vi "Run.vi"(8 "error in (no error)":errorcluster, 11 "Opctics in":refnum<class "Opt_Continuous.lvclass">) -> (0 "error out":errorcluster, 3 "Opt_Continuous out":refnum<class "Opt_Continuous.lvclass">)   [LabVIEW 2018, in "Opt_Continuous.lvclass"]
uses:
  Opt_Continuous.lvclass
  C:/Users/observer/Desktop/Sparc4GUI/SPARC4_GUI/Device/Optics/Optics.lvclass
  Optics.lvclass/Optics.ctl
  Optics.lvclass
  StateMachine/State Machine.lvclass
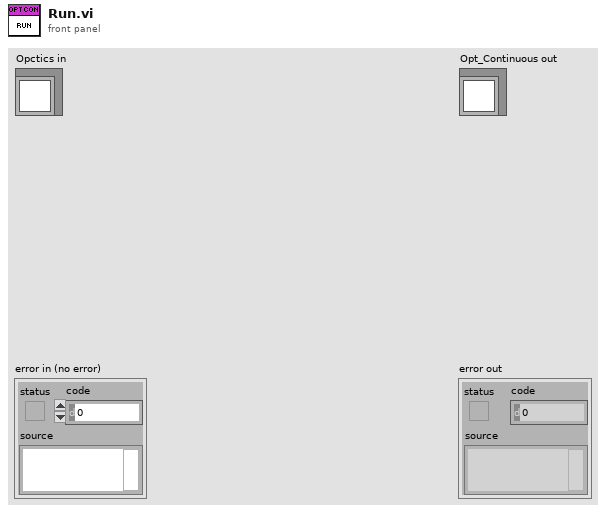
[diagram p1: front panel]
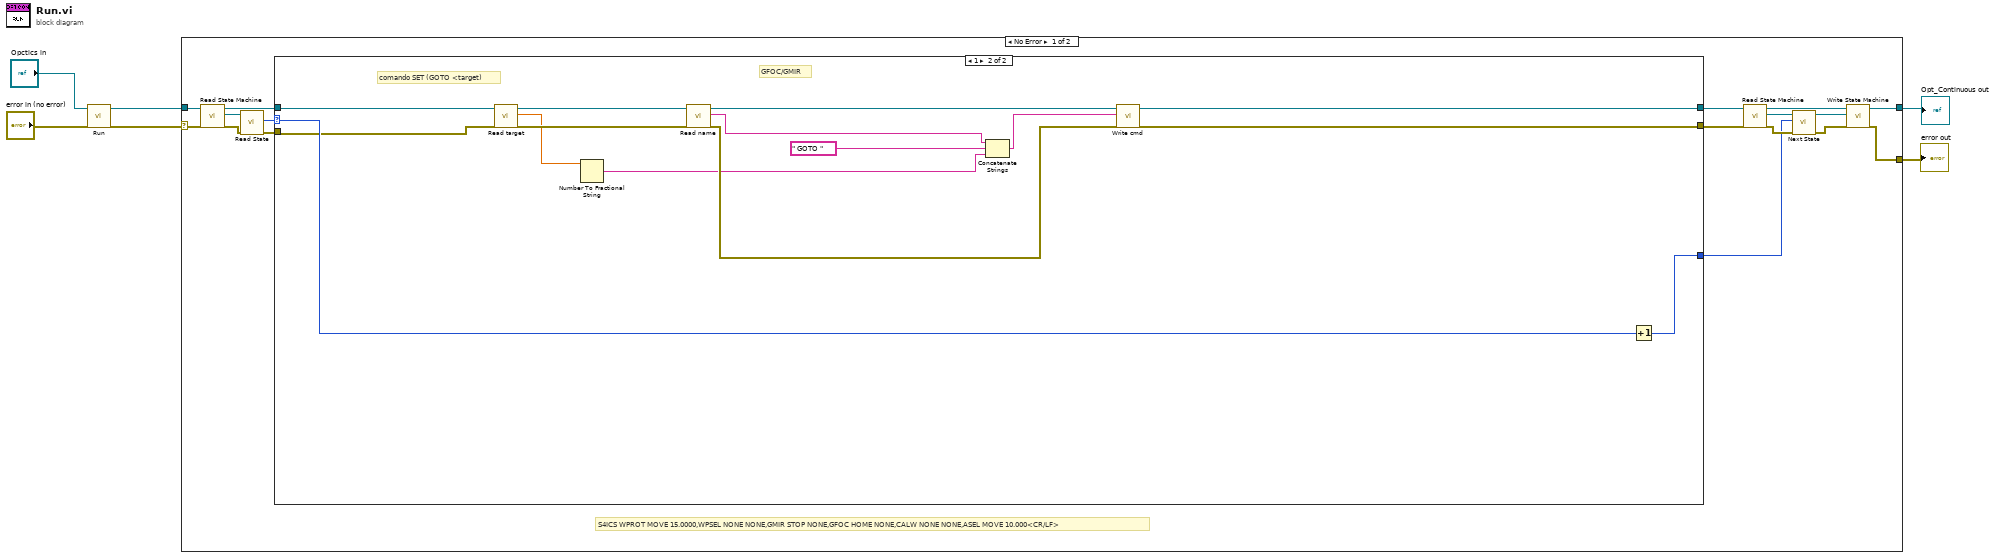
[diagram p0: block diagram]
diagram:
  n1 = call-parent "Run.vi"("error in (no error)"="error in (no error)", "Opctics in"="Opctics in") -> ("error out"=w4:errorcluster, "Optics out"=w3:refnum<class "Opt_Continuous.lvclass">)  [unwired: 8 in]
  n2 = case shown="No Error" w4 {
    selector: w4 -> [w22 w43]
    tunnel: [w7 w43] -> w1
    tunnel: [w12 w42] -> w2
    tunnel: w3 -> [w23 w42]
    frame No Error {
      # "S4ICS WPROT MOVE 15.0000,WPSEL NONE NONE,GMIR STOP NONE,GFOC HOME NONE,CALW NONE NONE,ASEL MOVE 10.000<CR/LF>"
      n3 = call-dynamic "Read State Machine.vi"("error in (no error)"=w22, "Device in"=w23) -> ("error out"=w19:errorcluster, "State Machine.lvclass"=w21:refnum<class "State Machine.lvclass">, "Device out"=w17:refnum<class "Opt_Continuous.lvclass">)  [unwired: 7 in]
      n4 = call-dynamic "Read State.vi"("error in (no error)"=w19, "State Machine in"=w21) -> ("error out"=w18:errorcluster, "State"=w20:i32)  [unwired: 7 in, 1 out]
      n5 = case shown="1" w20 {
        selector: w20 -> [w26 w37]
        tunnel: w18 -> [w24 w34]
        tunnel: [w24 w40] -> w8
        tunnel: w17 -> [w25 w35]
        tunnel: [w25 w41] -> w15
        tunnel: [w26 w38] -> w9
        frame Default {
        }
        frame 1 {
          # "GFOC/GMIR"
          # "comando SET (GOTO <target)"
          n6 = call "Read target.vi"("error in (no error)"=w34, "Optics in"=w35) -> ("error out"=w32:errorcluster, "target"=w28:dbl, "Optics out"=w30:refnum<class "Opt_Continuous.lvclass">)  [unwired: 7 in]
          n7 = Number To Fractional String(number=w28) -> (F-format string=w27:string)  [unwired: 3 in]
          n8 = call "Read name.vi"("error in (no error)"=w32, "Optics in"=w30) -> ("error out"=w31:errorcluster, "name"=w33:string, "Optics out"=w29:refnum<class "Opt_Continuous.lvclass">)  [unwired: 7 in]
          n9 = Concatenate Strings(w33, " GOTO " ("string"), w27) -> (w39:string)
          n10 = call-dynamic "Write cmd.vi"("error in (no error)"=w31, "cmd"=w39, "Device in"=w29) -> ("error out"=w40:errorcluster, "Device out"=w41:refnum<class "Opt_Continuous.lvclass">)  [unwired: 7 in]
          n11 = Increment(x=w37) -> (x+1=w38:i32)
        }
      }
      n12 = call-dynamic "Read State Machine.vi"("error in (no error)"=w8, "Device in"=w15) -> ("error out"=w11:errorcluster, "State Machine.lvclass"=w14:refnum<class "State Machine.lvclass">, "Device out"=w13:refnum<class "Opt_Continuous.lvclass">)  [unwired: 7 in]
      n13 = call "Next State.vi"("error in (no error)"=w11, "New_State"=w9, "State Machine in"=w14) -> ("error out"=w10:errorcluster, "State Machine out"=w16:refnum<class "State Machine.lvclass">)  [unwired: 7 in]
      n14 = call-dynamic "Write State Machine.vi"("error in (no error)"=w10, "State Machine.lvclass"=w16, "Device in"=w13) -> ("error out"=w7:errorcluster, "Device out"=w12:refnum<class "Opt_Continuous.lvclass">)  [unwired: 7 in]
    }
    frame Error {
    }
  }
  "error out" <- w1
  "Opt_Continuous out" <- w2
